vi "transmit.vi"() -> ()   [LabVIEW 2020]
uses:
  <vilib>/measure/NI_MABase.lvlib
panel:
  out "Package Directory":path
  out "Stop?":bool
  out "Terminal Output":string
  out "Transmitted Data":waveform(dbl)[](graph)
  out "Error Out":errorcluster
  in  "FMC Parameters":T1={"IP"="169.254.92.202", "Port"=22, "Username"="analog", "Password"="analog", "rfPort"="A", "Frequency"=2400, "Sample Rate"=30.72, "Bandwidth"=18, "Tx Attenuation"=0, "Cyclic?"=TRUE}
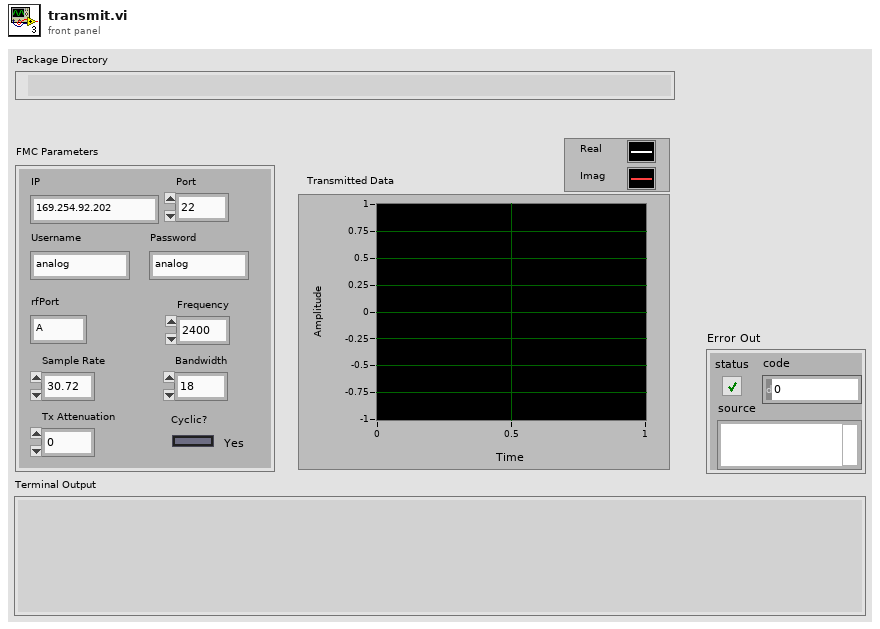
[diagram p1: front panel]
types:
  T1 = cluster{"IP":string, "Port":i32, "Username":string, "Password":string, "rfPort":string, "Frequency":i64, "Sample Rate":dbl, "Bandwidth":i32, "Tx Attenuation":i32, "Cyclic?":bool}
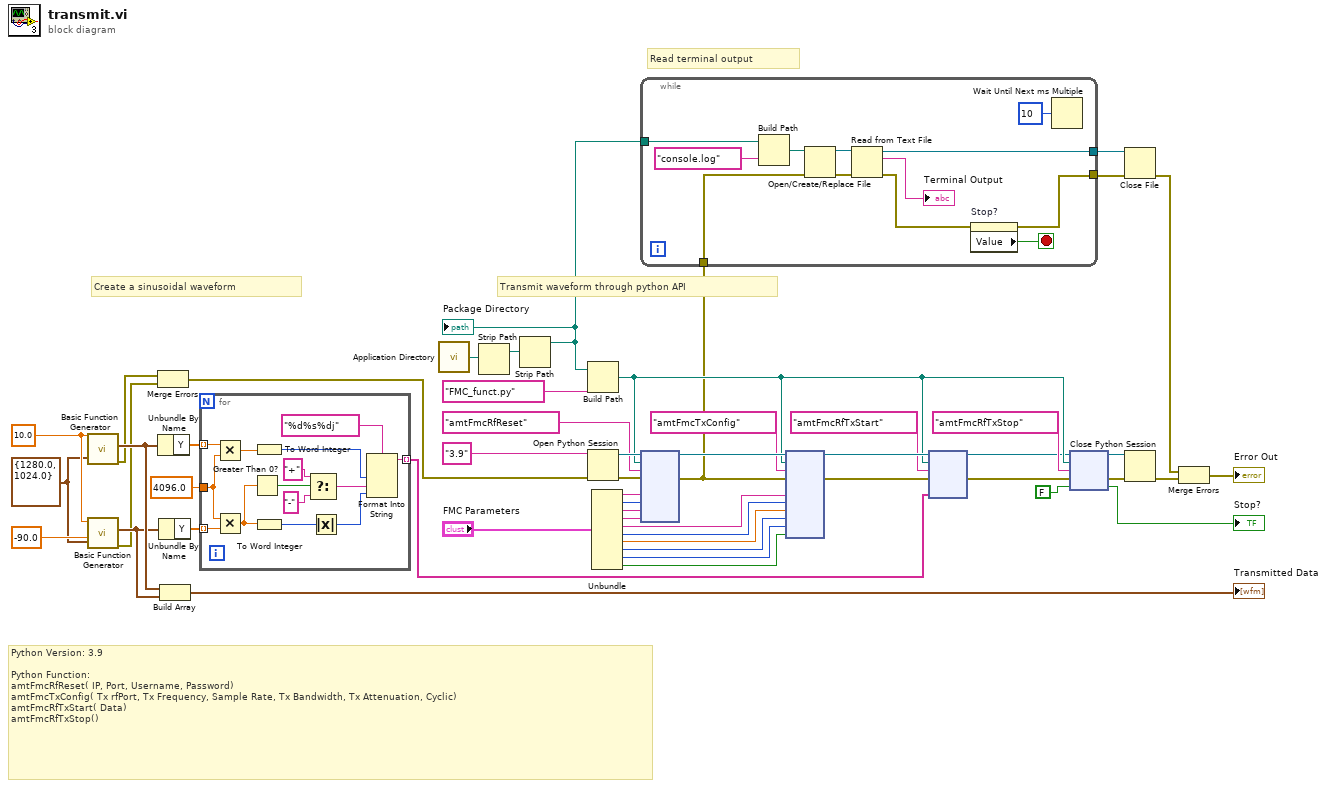
[diagram p0: block diagram]
diagram:
  w46 = 10.0 ("frequency")
  w44 = cluster{"Fs":dbl, "#s":dbl} {"Fs"=1280.0, "#s"=1024.0} ("sampling info")
  # "Read terminal output"
  # "Python Version: 3.9\n\nPython Function:\namtFmcRfReset( IP, Port, Username, Password)\namtFmcTxConfig( Tx rfPort, Tx Frequency, Sample Rate, Tx Bandwidth, Tx Attenuation, Cyclic)\namtFmcRfTxStart( Data)\namtFmcRfTxStop()"
  # "Create a sinusoidal waveform"
  # "Transmit waveform through python API"
  n1 = call <vilib>:"Basic Function Generator.vi"("sampling info"=w44, "frequency"=w46) -> ("error out"=w2:errorcluster, "signal out"=w40:waveform(dbl))  [unwired: 7 in, 1 out]
  n2 = call <vilib>:"Basic Function Generator.vi"("sampling info"=w44, "phase"=-90.0, "frequency"=w46) -> ("error out"=w3:errorcluster, "signal out"=w39:waveform(dbl))  [unwired: 6 in, 1 out]
  n3 = Merge Errors(w2, w3) -> (w1:errorcluster)
  n4 = Unbundle By Name(w40) -> ("Y"=w42:dbl[])
  n5 = Unbundle By Name(w39) -> ("Y"=w41:dbl[])
  n6 = Build Array(w40, w39) -> (→"Transmitted Data":waveform(dbl)[])
  n7 = for {
    tunnel: w41 -> [w65] mode=indexing
    tunnel: w42 -> [w64] mode=indexing
    tunnel: 4096.0 -> [w63]
    tunnel: [w54] -> w19 mode=indexing
    n8 = Multiply(x=w64, y=w63) -> (x*y=w61:dbl)
    n9 = Multiply(x=w63, y=w65) -> (x*y=w60:dbl)
    n10 = Greater Than 0?(x=w60) -> (x > 0?=w62:bool)
    n11 = To Word Integer(number=w61) -> (16bit integer=w58:i16)
    n12 = To Word Integer(number=w60) -> (16bit integer=w52:i16)
    n13 = Select(t="+", s=w62, f="-") -> (s? t:f=w59:string)
    n14 = Absolute Value(x=w52) -> (abs(x)=w53:i16)
    n15 = Format Into String(format string="%d%s%dj", w58, w59, w53) -> (resulting string=w54:string)  [unwired: 2 in, 1 out]
  }
  n16 = call <vilib>:"Application Directory.vi"() -> ("Application Directory"=w6:path)
  n17 = Strip Path(path=w6) -> (stripped path=w5:path)  [unwired: 1 out]
  n18 = Strip Path(path=w5) -> (stripped path=w4:path)  [unwired: 1 out]
  "Package Directory" <- w4
  n19 = Build Path(base path=w4, name or relative path="FMC_funct.py") -> (appended path=w33:path)
  n20 = Open Python Session(python version="3.9" ("Python version"), 3:w1) -> (session out=w50:refnum<k35>, error out=w51:errorcluster)  [unwired: 1 in]
  n21 = Unbundle("FMC Parameters") -> ("IP"=w29:string, "Port"=w28:i32, "Username"=w27:string, "Password"=w26:string, "rfPort"=w25:string, "Frequency"=w24:i64, "Sample Rate"=w23:dbl, "Bandwidth"=w22:i32, "Tx Attenuation"=w21:i32, "Cyclic?"=w20:bool)
  n22 = node(w50, w33, "amtFmcRfReset" ("function name"), w51, w29, w28, w27, w26) -> (w36:refnum<k35>, w16:errorcluster)  [unwired: 6 in, 2 out]
  n23 = while {
    tunnel: w4 -> [w72]
    tunnel: w16 -> [w71]
    tunnel: [w68] -> w13
    tunnel: [w66] -> w12
    stop <- w69 stop-if-true
    n24 = Build Path(base path=w72, name or relative path="console.log" ("function name")) -> (appended path=w77:path)
    n25 = Open/Create/Replace File(file path (use dialog)=w77, error in=w71) -> (refnum out=w74:refnum<file>, error out=w75:errorcluster)  [unwired: 4 in, 1 out]
    n26 = Read from Text File(file (use dialog)=w74, error in=w75) -> (refnum out=w66:refnum<file>, text=→"Terminal Output":string, error out=w67:errorcluster)  [unwired: 2 in, 1 out]
    n27 = property on="Stop?" class="Bool (strict)"(error in=w67) -> (error out=w68:errorcluster, "Value"=w69:bool)  [unwired: 1 in, 1 out]
    n28 = Wait Until Next ms Multiple(millisecond multiple=u32 10) -> ()  [unwired: 1 out]
  }
  n29 = node(w36, w33, "amtFmcTxConfig" ("function name"), w16, w25, w24, w23, w22, w21, w20) -> (w35:refnum<k35>, w30:errorcluster)  [unwired: 8 in, 2 out]
  n30 = node(w35, w33, "amtFmcRfTxStart" ("function name"), w30, w19) -> (w10:refnum<k35>, w11:errorcluster)  [unwired: 3 in, 2 out]
  n31 = node(w10, w33, "amtFmcRfTxStop" ("function name"), w11, FALSE) -> (w17:refnum<k35>, w18:errorcluster, →"Stop?":bool)  [unwired: 2 out]
  n32 = Close File(refnum=w12, error in=w13) -> (error out=w9:errorcluster)  [unwired: 1 out]
  n33 = Close Python Session(session in=w17, error in=w18) -> (11:w8:errorcluster)
  n34 = Merge Errors(w9, w8) -> (→"Error Out":errorcluster)
